vi "Configure Digital Channel.vi"(7 "Enable Channel (T:Enable)":bool, 8 "error in (no error)":errorcluster, 9 "Threshold (1.4)":dbl, 10 "Channel (13 : Digital 0)":i32(ring) items=["Digital 0", "Digital 1", "Digital 2", "Digital 3", "Digital 4", "Digital 5", "Digital 6", "Digital 7", "Digital 8", "Digital 9", "Digital 10", "Digital 11", "Digital 12", "Digital 13", "Digital 14", "Digital 15", "POD1", "POD2"], 11 "VISA resource name":refnum<visa-resource-name>) -> (0 "error out":errorcluster, 3 "VISA resource name out":refnum<visa-resource-name>)   [LabVIEW 2009, in "Agilent 8000 Series.lvlib"]
doc: "Configures the common properties of the oscilloscope's digtial channel subsystem for a particular channel. These properties are Threshold and channel enabled."
uses:
  Agilent 8000 Series.lvlib
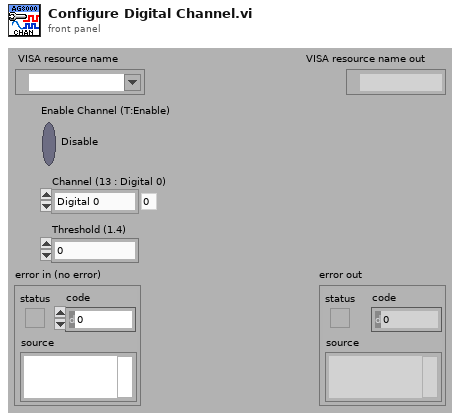
[diagram p1: front panel]
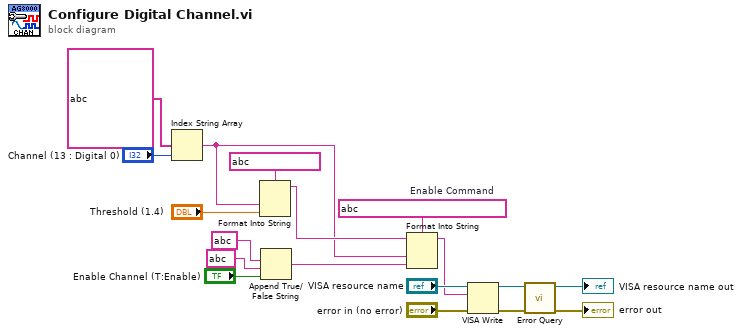
[diagram p0: block diagram]
diagram:
  w2 = string ?  # Enable Command
  n1 = Index String Array(1:"Channel (13 : Digital 0)", 2:string[] ?) -> (0:w3:string)  [unwired: 1 in]
  n2 = Format Into String(format string=string ?, w3, "Threshold (1.4)") -> (resulting string=w4:string)  [unwired: 2 in, 1 out]
  n3 = Append True/False String(1:"Enable Channel (T:Enable)", 2:string ? ("false string"), 3:string ? ("true string")) -> (0:w5:string)  [unwired: 1 in]
  n4 = Format Into String(format string=w2, initial string=w4, w3, w5) -> (resulting string=w1:string)  [unwired: 1 in, 1 out]
  n5 = VISA Write(VISA resource name="VISA resource name", write buffer=w1, error in (no error)="error in (no error)") -> (VISA resource name out=w14:refnum<visa-resource-name>, error out=w13:errorcluster)  [unwired: 1 out]
  n6 = call "Error Query.vi"("error in (no error)"=w13, "VISA resource name"=w14) -> ("error out"=→"error out":errorcluster, "VISA resource name out"=→"VISA resource name out":refnum<visa-resource-name>)  [unwired: 6 in, 2 out]
